vi "LogEvent.vi"(8 "error in (no error)":errorcluster, 9 "eventInfo":dbl=nan, 10 "Event Name":string="acquireFixation", 11 "TrialBasedExperiment in":refnum<class "TrialBasedExperiment.lvclass">) -> (0 "error out":errorcluster, 3 "TrialBasedExperiment out":refnum<class "TrialBasedExperiment.lvclass">)   [LabVIEW 2010, in "TrialBasedExperiment.lvclass"]
uses:
  TrialBasedExperiment.lvclass
  Core SubVIs/Core SubVIs.lvlib
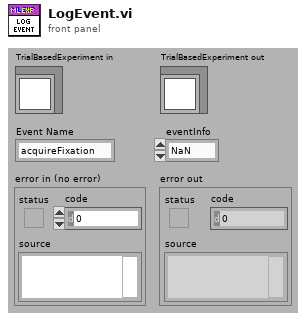
[diagram p1: front panel]
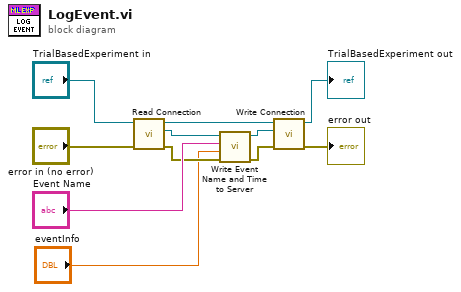
[diagram p0: block diagram]
diagram:
  n1 = call-dynamic "Read Connection.vi"("error in (no error)"="error in (no error)", "TrialBasedExperiment in"="TrialBasedExperiment in") -> ("error out"=w3:errorcluster, "Connection"=w7:refnum<k5>, "TrialBasedExperiment out"=w5:refnum<class "TrialBasedExperiment.lvclass">)  [unwired: 7 in]
  n2 = call "Write Event Name and Time to Server.vi"("error in (no error)"=w3, "eventInfo"="eventInfo", "Event Name"="Event Name", "connection ID"=w7) -> ("error out"=w2:errorcluster, "connection ID duplicate"=w6:refnum<k5>)  [unwired: 6 out]
  n3 = call-dynamic "Write Connection.vi"("error in (no error)"=w2, "Connection"=w6, "TrialBasedExperiment in"=w5) -> ("error out"=→"error out":errorcluster, "TrialBasedExperiment out"=→"TrialBasedExperiment out":refnum<class "TrialBasedExperiment.lvclass">)  [unwired: 7 in]
